vi "数据测量区转CDAB.vi"(11 "测量数据区":T1 {"单位" items=["ug/L", "mg/L", "ppm", "mg/m3", "cm", "ppb", "ug/m3", "%", "nmol/mol", "umol/mol", "MPN/L", "MPN/100ml", "ng/m3", "NTU", "无量纲", "ms/cm", "us/cm", "℃", "mV", "万个/L"]}) -> (3 "输出数组":u16[](array[numeric]))   [LabVIEW 2016]
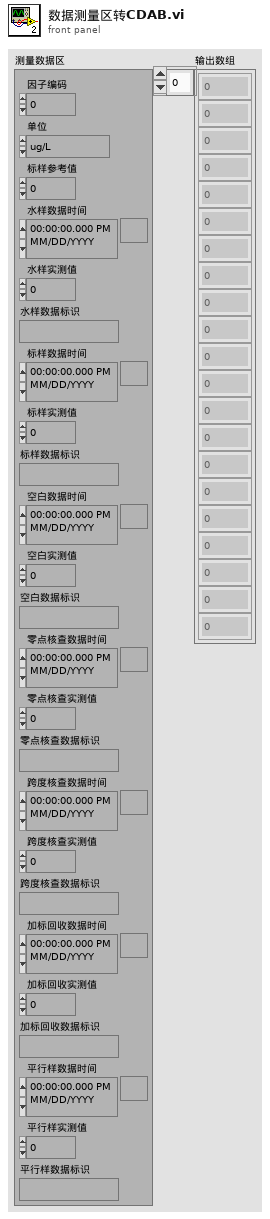
[diagram p1: front panel]
types:
  T1 = cluster{"因子编码":u32, "单位":u16, "标样参考值":sgl, "水样数据时间":timestamp, "水样实测值":sgl, "水样数据标识":string, "标样数据时间":timestamp, "标样实测值":sgl, "标样数据标识":string, "空白数据时间":timestamp, "空白实测值":sgl, "空白数据标识":string, "零点核查数据时间":timestamp, "零点核查实测值":sgl, "零点核查数据标识":string, "跨度核查数据时间":timestamp, "跨度核查实测值":sgl, "跨度核查数据标识":string, "加标回收数据时间":timestamp, "加标回收实测值":sgl, "加标回收数据标识":string, "平行样数据时间":timestamp, "平行样实测值":sgl, "平行样数据标识":string}
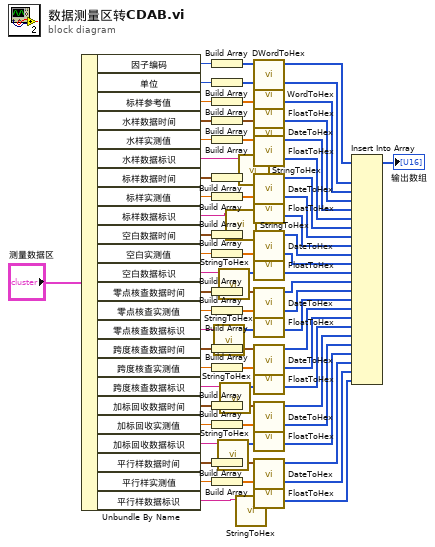
[diagram p0: block diagram]
diagram:
  n1 = Unbundle By Name("测量数据区") -> ("因子编码"=w66:u32, "单位"=w64:u16, "标样参考值"=w59:sgl, "水样数据时间"=w58:timestamp, "水样实测值"=w60:sgl, "水样数据标识"=w15:string, "标样数据时间"=w54:timestamp, "标样实测值"=w57:sgl, "标样数据标识"=w12:string, "空白数据时间"=w53:timestamp, "空白实测值"=w56:sgl, "空白数据标识"=w8:string, "零点核查数据时间"=w52:timestamp, "零点核查实测值"=w55:sgl, "零点核查数据标识"=w11:string, "跨度核查数据时间"=w51:timestamp, "跨度核查实测值"=w50:sgl, "跨度核查数据标识"=w10:string, "加标回收数据时间"=w49:timestamp, "加标回收实测值"=w48:sgl, "加标回收数据标识"=w9:string, "平行样数据时间"=w47:timestamp, "平行样实测值"=w46:sgl, "平行样数据标识"=w3:string)
  n2 = Build Array(w66) -> (w61:u32[])
  n3 = Build Array(w64) -> (w63:u16[])
  n4 = Build Array(w59) -> (w45:sgl[])
  n5 = Build Array(w58) -> (w38:timestamp[])
  n6 = Build Array(w60) -> (w30:sgl[])
  n7 = Build Array(w54) -> (w32:timestamp[])
  n8 = Build Array(w57) -> (w31:sgl[])
  n9 = Build Array(w53) -> (w43:timestamp[])
  n10 = Build Array(w56) -> (w37:sgl[])
  n11 = Build Array(w52) -> (w42:timestamp[])
  n12 = Build Array(w55) -> (w36:sgl[])
  n13 = Build Array(w51) -> (w41:timestamp[])
  n14 = Build Array(w50) -> (w35:sgl[])
  n15 = Build Array(w49) -> (w40:timestamp[])
  n16 = Build Array(w48) -> (w34:sgl[])
  n17 = Build Array(w47) -> (w39:timestamp[])
  n18 = Build Array(w46) -> (w33:sgl[])
  n19 = call "StringToHex.vi"("字符串"=w11) -> ("数组"=w6:u16[])  [unwired: 10 in]
  n20 = call "StringToHex.vi"("字符串"=w9) -> ("数组"=w2:u16[])  [unwired: 10 in]
  n21 = call "StringToHex.vi"("字符串"=w8) -> ("数组"=w7:u16[])  [unwired: 10 in]
  n22 = call "StringToHex.vi"("字符串"=w10) -> ("数组"=w5:u16[])  [unwired: 10 in]
  n23 = call "StringToHex.vi"("字符串"=w12) -> ("数组"=w13:u16[])  [unwired: 10 in]
  n24 = call "StringToHex.vi"("字符串"=w3) -> ("数组"=w4:u16[])  [unwired: 10 in]
  n25 = call "StringToHex.vi"("字符串"=w15) -> ("数组"=w14:u16[])  [unwired: 10 in]
  n26 = call "DWordToHex.vi"("DWORD"=w61) -> ("数组"=w65:u16[])  [unwired: 10 in]
  n27 = call "WordToHex.vi"("WORD"=w63) -> ("数组"=w62:u16[])  [unwired: 10 in]
  n28 = call "FloatToHex.vi"("浮点数"=w45) -> ("DCBA整形输出"=w44:u16[])  [unwired: 10 in]
  n29 = call "DateToHex.vi"("DATE"=w38) -> ("数组"=w29:u16[])  [unwired: 10 in]
  n30 = call "FloatToHex.vi"("浮点数"=w30) -> ("DCBA整形输出"=w28:u16[])  [unwired: 10 in]
  n31 = call "DateToHex.vi"("DATE"=w32) -> ("数组"=w16:u16[])  [unwired: 10 in]
  n32 = call "FloatToHex.vi"("浮点数"=w31) -> ("DCBA整形输出"=w27:u16[])  [unwired: 10 in]
  n33 = call "DateToHex.vi"("DATE"=w43) -> ("数组"=w26:u16[])  [unwired: 10 in]
  n34 = call "FloatToHex.vi"("浮点数"=w37) -> ("DCBA整形输出"=w25:u16[])  [unwired: 10 in]
  n35 = call "DateToHex.vi"("DATE"=w42) -> ("数组"=w24:u16[])  [unwired: 10 in]
  n36 = call "FloatToHex.vi"("浮点数"=w36) -> ("DCBA整形输出"=w23:u16[])  [unwired: 10 in]
  n37 = call "DateToHex.vi"("DATE"=w41) -> ("数组"=w22:u16[])  [unwired: 10 in]
  n38 = call "FloatToHex.vi"("浮点数"=w35) -> ("DCBA整形输出"=w21:u16[])  [unwired: 10 in]
  n39 = call "DateToHex.vi"("DATE"=w40) -> ("数组"=w20:u16[])  [unwired: 10 in]
  n40 = call "FloatToHex.vi"("浮点数"=w34) -> ("DCBA整形输出"=w19:u16[])  [unwired: 10 in]
  n41 = call "DateToHex.vi"("DATE"=w39) -> ("数组"=w18:u16[])  [unwired: 10 in]
  n42 = call "FloatToHex.vi"("浮点数"=w33) -> ("DCBA整形输出"=w17:u16[])  [unwired: 10 in]
  n43 = Insert Into Array(array=w65, new element #1=w62, new element #2=w44, new element #3=w29, new element #4=w28, new element #5=w14, new element #6=w16, new element #7=w27, new element #8=w13, new element #9=w26, new element #10=w25, new element #11=w7, new element #12=w24, new element #13=w23, new element #14=w6, new element #15=w22, new element #16=w21, new element #17=w5, new element #18=w20, new element #19=w19, new element #20=w2, new element #21=w18, new element #22=w17, new element #23=w4) -> (→"输出数组":u16[])  [unwired: 1 in]
